vi "BRig_RT__Case_Idle__State_DispenseWater_Delay.vi"(9 "input_increment":i64, 10 "input_state":T1, 11 "input_dataMTrig":u16[](array[numeric])) -> (2 "output_state":T1, 3 "output_dataMTrig":u16[](array[numeric]))   [LabVIEW 2014]
uses:
  myRIO_Gil_RT__stateList_7,4__NoExp.ctl
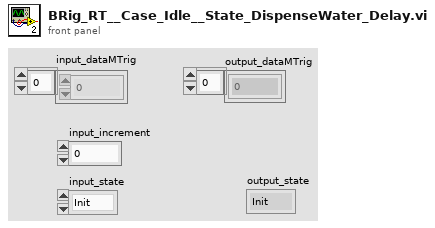
[diagram p1: front panel]
types:
  T1 = typedef "myRIO_Gil_RT__stateList_7,4__NoExp.ctl" = enum16{"Init", "UploadSettings", "Idle", "RewardCalibration_pre", "DispenseWater_pre", "DispenseWater", "DispenseWater_Delay_pre", "DispenseWater_Delay", "TestConnection", "End"}
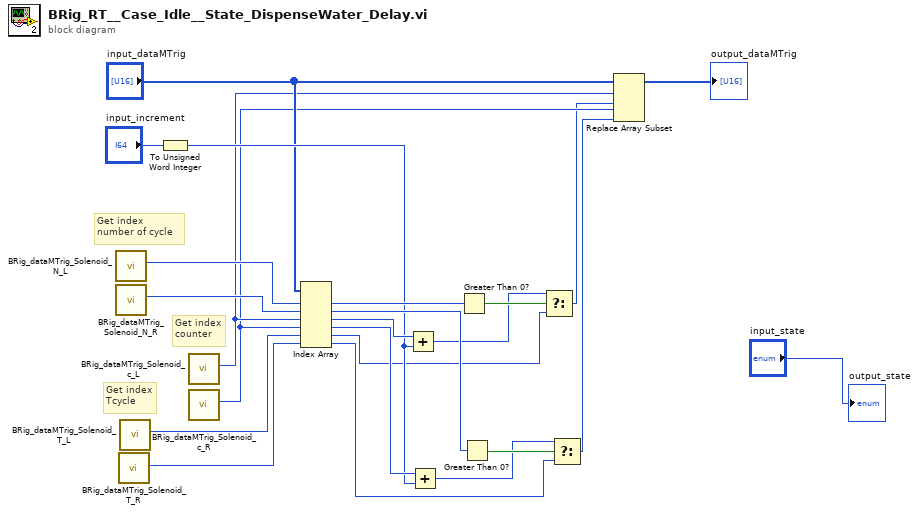
[diagram p0: block diagram]
diagram:
  # "Get index\nTcycle"
  # "Get index\nnumber of cycle"
  # "Get index\ncounter"
  n1 = call "BRig_dataMTrig_Solenoid_N_L.vi"() -> ("output_Solenoid_N_L"=w23:i32)  [unwired: 11 in]
  n2 = call "BRig_dataMTrig_Solenoid_N_R.vi"() -> ("output_Solenoid_N__R"=w22:i32)  [unwired: 11 in]
  n3 = call "BRig_dataMTrig_Solenoid_T_R.vi"() -> ("output_Solenoid_T_R"=w20:i32)  [unwired: 11 in]
  n4 = call "BRig_dataMTrig_Solenoid_T_L.vi"() -> ("output_Solenoid_T_L"=w21:i32)  [unwired: 11 in]
  n5 = To Unsigned Word Integer(number="input_increment") -> (unsigned 16bit integer=w14:u16)
  n6 = call "BRig_dataMTrig_Solenoid_c_L.vi"() -> ("output_Solenoid_c_L"=w5:i32)  [unwired: 11 in]
  n7 = call "BRig_dataMTrig_Solenoid_c_R.vi"() -> ("output_Solenoid_c_R"=w4:i32)  [unwired: 11 in]
  n8 = Index Array(array="input_dataMTrig", index #1=w23, index #2=w22, index #3=w5, index #4=w4, index #5=w21, index #6=w20) -> (element #1=w19:u16, element #2=w18:u16, element #3=w16:u16, element #4=w15:u16, element #5=w9:u16, element #6=w8:u16)
  n9 = Add(x=w16, y=w14) -> (x+y=w12:u16)
  n10 = Add(x=w15, y=w14) -> (x+y=w10:u16)
  n11 = Greater Than 0?(x=w19) -> (x > 0?=w13:bool)
  n12 = Greater Than 0?(x=w18) -> (x > 0?=w11:bool)
  n13 = Select(t=w12, s=w13, f=w9) -> (s? t:f=w3:u16)
  n14 = Select(t=w10, s=w11, f=w8) -> (s? t:f=w2:u16)
  n15 = Replace Array Subset(array="input_dataMTrig", new element #1=w3, index #1=w5, new element #2=w2, index #2=w4) -> (→"output_dataMTrig":u16[])
  "output_state" <- "input_state"
